vi "Reset.vi"(0 "VISA resource name":refnum<visa-resource-name>, 11 "error in (no error)":errorcluster) -> (4 "VISA resource name out":refnum<visa-resource-name>, 15 "error out":errorcluster)   [LabVIEW 2013]
doc: "This VI resets the instrument, and then sends a set of default setup commands to the instrument."
uses:
  <instrlib>/Yokogawa WT200 Series/Yokogawa WT200 Series.lvlib
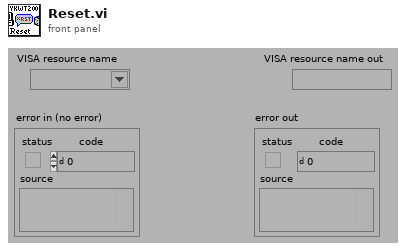
[diagram p1: front panel]
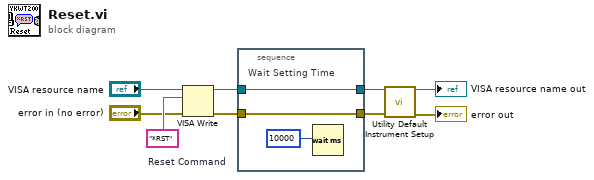
[diagram p0: block diagram]
diagram:
  w9 = "*RST"  # Reset Command
  n1 = VISA Write(VISA resource name="VISA resource name", write buffer=w9, error in (no error)="error in (no error)") -> (VISA resource name out=w2:refnum<visa-resource-name>, error out=w4:errorcluster)  [unwired: 1 out]
  n2 = stacked-sequence {
    tunnel: w4 -> [w11]
    tunnel: [w11] -> w3
    tunnel: w2 -> [w10]
    tunnel: [w10] -> w1
    frame #0 {
      # "Wait Setting Time"
      n3 = Wait (ms)(milliseconds to wait=u32 10000) -> ()  [unwired: 1 out]
    }
  }
  n4 = call <instrlib>:"Utility Default Instrument Setup.vi"("VISA resource name"=w1, "error in (no error)"=w3) -> ("VISA resource name out"=→"VISA resource name out":refnum<visa-resource-name>, "error out"=→"error out":errorcluster)  [unwired: 12 in]
